vi "Remove Timer.vi"(10 "Name":string, 11 "UserEventTimer in":refnum<class "TimerEngine.lvclass">) -> (3 "UserEventTimer out":refnum<class "TimerEngine.lvclass">)   [LabVIEW 2017, in "TimerEngine.lvlib" / "TimerEngine.lvclass"]
uses:
  TimerEngine.lvclass
  TimerEngine.lvclass/TimerEngine.ctl
  _TimerClass/Timer.lvclass/Timer.ctl
  _TimerClass/Timer.lvclass
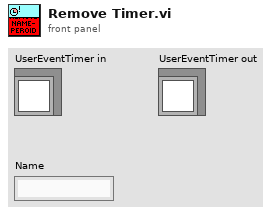
[diagram p1: front panel]
types:
  T1 = typedef "TimerEngine.lvlib/TimerEngine.lvclass/Timer-UserEvent.ctl" = refnum<user-event>
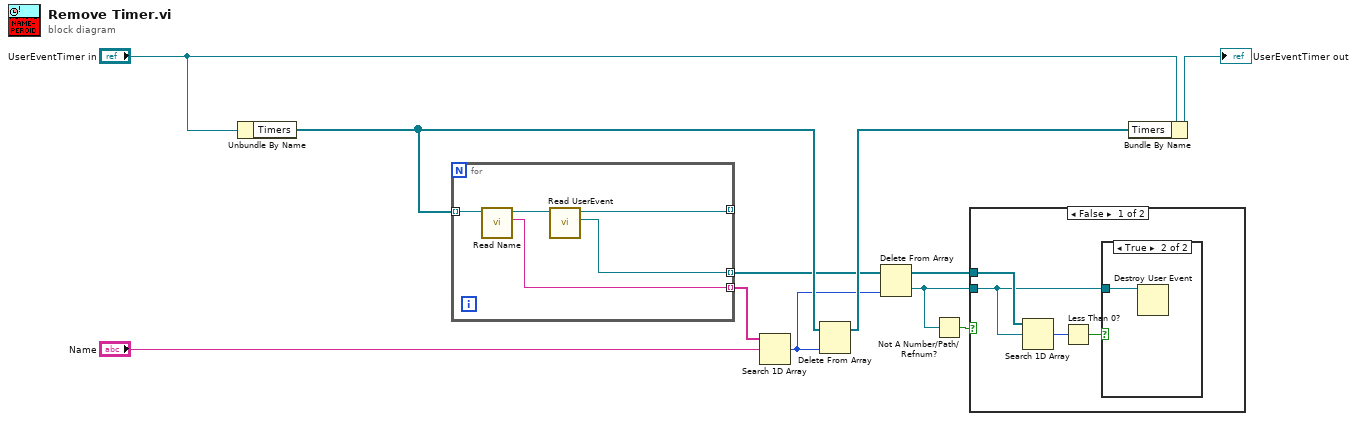
[diagram p0: block diagram]
diagram:
  n1 = Unbundle By Name("UserEventTimer in") -> ("Timers"=w7:refnum<class "Timer.lvclass">[])
  n2 = for {
    tunnel: w7 -> [w16] mode=indexing
    tunnel: [w13] -> _ mode=indexing
    tunnel: [w14] -> w6 mode=indexing
    tunnel: [w12] -> w5 mode=indexing
    n3 = call "Read Name.vi"("Timer in"=w16) -> ("Name"=w14:string, "Timer out"=w15:refnum<class "Timer.lvclass">)  [unwired: 8 in, 1 out]
    n4 = call "Read UserEvent.vi"("Timer in"=w15) -> ("UserEvent"=w12:T1, "Timer out"=w13:refnum<class "Timer.lvclass">)  [unwired: 8 in, 1 out]
  }
  n5 = Search 1D Array(1D array=w6, element="Name") -> (index of element=w4:i32)  [unwired: 1 in]
  n6 = Delete From Array(array=w7, index=w4) -> (array with subset deleted=w8:refnum<class "Timer.lvclass">[])  [unwired: 1 in, 1 out]
  n7 = Delete From Array(array=w5, index=w4) -> (deleted portion=w2:T1, array with subset deleted=w3:T1[])  [unwired: 1 in]
  n8 = Not A Number/Path/Refnum?(number/path/refnum=w2) -> (NaN/Path/Refnum?=w1:bool)
  n9 = case shown="False" w1 {
    tunnel: w3 -> [w18 _]
    tunnel: w2 -> [w17 _]
    frame False {
      n10 = Search 1D Array(1D array=w18, element=w17) -> (index of element=w20:i32)  [unwired: 1 in]
      n11 = Less Than 0?(x=w20) -> (x < 0?=w19:bool)
      n12 = case shown="True" w19 {
        tunnel: w17 -> [_ w21]
        frame False {
        }
        frame True {
          n13 = Destroy User Event(user event=w21) -> ()  [unwired: 1 in, 1 out]
        }
      }
    }
    frame True {
    }
  }
  n14 = Bundle By Name(cluster="UserEventTimer in", "Timers"=w8) -> (→"UserEventTimer out":refnum<class "TimerEngine.lvclass">)
